vi "delay.vi"(8 "error in":errorcluster caption="error in (no error)", 10 "Milliseconds to wait":i32=50, 11 "VISA resource name":refnum<visa-resource-name>) -> (0 "error out":errorcluster, 3 "VISA resource name out":refnum<visa-resource-name>)   [LabVIEW 2020, in "Rohde&Schwarz RTx Oscilloscopes.lvlib" / "rsidr_core.lvlib"]
uses:
  rsidr_core.lvlib
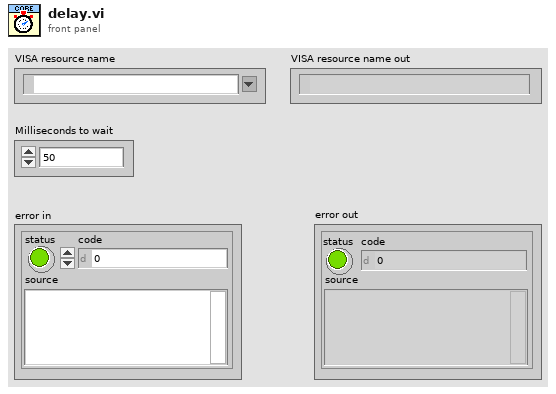
[diagram p1: front panel]
types:
  T1 = typedef "Rohde&Schwarz RTx Oscilloscopes.lvlib/rsidr_core.lvlib/type_Session_Data.ctl" = cluster{"IDN string":string, "Instrument FW":string, "Instr type":string, "Instr type for err. msg.":string, "Installed Options":string[], "Ignore Error Messages":string, "Logging params":variant, "OPC Timeout":i32, "VISA Timeout":i32, "STB Poll VISA Timeout":i32, "Additional Flags":i32, "Wait Before Read":i32, "Wait Before Write":i32, "Option String Flags":i32, "IO Segment Size":i64, "VISA Access Mode":T2, "Interface Type":T3, "OPC Wait Mode":T4, "Bin Float Number  Format":T5, "Bin Integer Number Format":T6, "Simulate":bool, "VXIcapable":bool, "Duplicate Session":bool, "Add LF to Write":bool, "Logging":bool, "Fast Sweep":bool, "Query Instrument Status":bool, "Check Range":bool, "Check Options":bool, "OPC-sync Attr Writes":bool, "OPC-sync Attr Queries":bool}
  T2 = typedef "Rohde&Schwarz RTx Oscilloscopes.lvlib/rsidr_core.lvlib/type_VisaAccessMode.ctl" = u16
  T3 = typedef "Rohde&Schwarz RTx Oscilloscopes.lvlib/rsidr_core.lvlib/type_InterfaceType.ctl" = enum16{"Unknown", "GPIB", "VXI", "GPIB_VXI", "ASRL", "PXI", "TCPIP", "USB", "SOCKET"}
  T4 = typedef "Rohde&Schwarz RTx Oscilloscopes.lvlib/rsidr_core.lvlib/type_OPC_Wait_Mode.ctl" = enum16{"STBpolling", "STBpollingSlow", "STBpollingSuperSlow", "ServiceRequest", "OPCquery"}
  T5 = typedef "Rohde&Schwarz RTx Oscilloscopes.lvlib/rsidr_core.lvlib/type_Binary_Float_Number_Format.ctl" = enum16{"Float_4_Bytes_Swapped", "Float_4_Bytes", "Double_8_Bytes_Swapped", "Double_8_Bytes"}
  T6 = typedef "Rohde&Schwarz RTx Oscilloscopes.lvlib/rsidr_core.lvlib/type_Binary_Integer_Number_Format.ctl" = enum16{"Int32_4_Bytes_Swapped", "Int32_4 Bytes", "Int16_2_Bytes_Swapped", "Int16_2_Bytes"}
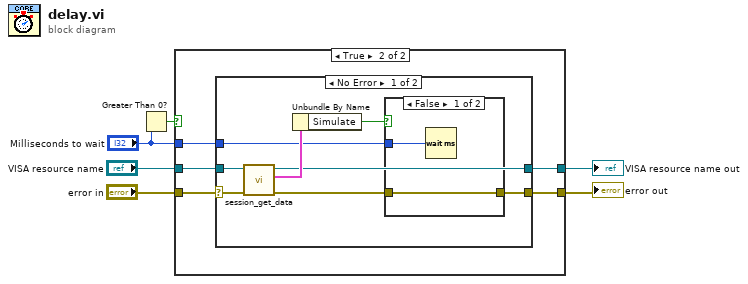
[diagram p0: block diagram]
diagram:
  n1 = Greater Than 0?(x="Milliseconds to wait") -> (x > 0?=w2:bool)
  n2 = case shown="True" w2 {
    tunnel: [w8 w13] -> w6
    tunnel: "VISA resource name" -> [w7 w12]
    tunnel: "error in" -> [w8 w11]
    tunnel: "Milliseconds to wait" -> [_ w10]
    tunnel: [w7 w9] -> w1
    frame False {
    }
    frame True {
      n3 = case shown="No Error" w11 {
        selector: w11 -> [w20 w26]
        tunnel: [w21 w26] -> w13
        tunnel: w12 -> [w19 w25]
        tunnel: w10 -> [w15 _]
        tunnel: [w14 w25] -> w9
        frame No Error {
          n4 = call "session_get_data.vi"("error in"=w20, "VISA resource name"=w19) -> ("error out"=w18:errorcluster, "Session User Data out"=w17:T1, "VISA resource name out"=w14:refnum<visa-resource-name>)  [unwired: 6 in, 1 out]
          n5 = Unbundle By Name(w17) -> ("Simulate"=w16:bool)
          n6 = case shown="False" w16 {
            tunnel: [w23 w24] -> w21
            tunnel: w18 -> [w23 w24]
            tunnel: w15 -> [w22 _]
            frame False {
              n7 = Wait (ms)(milliseconds to wait=w22) -> ()  [unwired: 1 out]
            }
            frame True {
            }
          }
        }
        frame Error {
        }
      }
    }
  }
  "VISA resource name out" <- w1
  "error out" <- w6
